vi "Configure Modulation(Phase).vi"(0 "VISA resource name":refnum<visa-resource-name>, 1 "Enable Phase Modulation (F: Disable)":bool, 2 "Phase Deviation (90 Degree)":dbl=90.0, 5 "Channel (1: Channel 1)":i32(ring)=1 items=["Channel 1"=1, "Channel 2"=2], 7 "PM Source (0: Internal)":i32(ring) items=["Internal", "External"], 9 "Modulation Waveform (0: Sinusoid)":i32(ring) items=["Sinusoid", "Square", "Triangle", "Ramp", "Nramp", "Noise", "User"], 11 "error in (no error)":errorcluster, 12 "Modulation Frequency (100 Hz)":dbl=100.0) -> (4 "VISA resource name out":refnum<visa-resource-name>, 15 "error out":errorcluster)   [LabVIEW 2012, in "RIGOL DG4000 Series.lvlib"]
doc: "Configures phase modulation."
uses:
  <instrlib>/RIGOL DG4000 Series/RIGOL DG4000 Series.lvlib
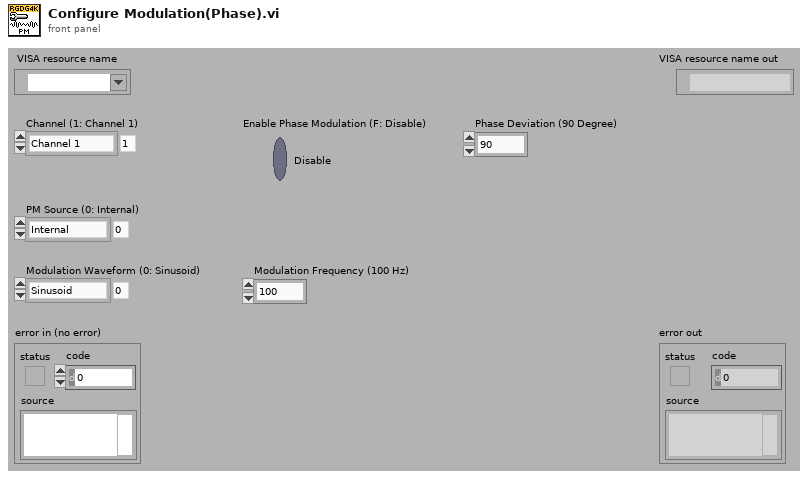
[diagram p1: front panel]
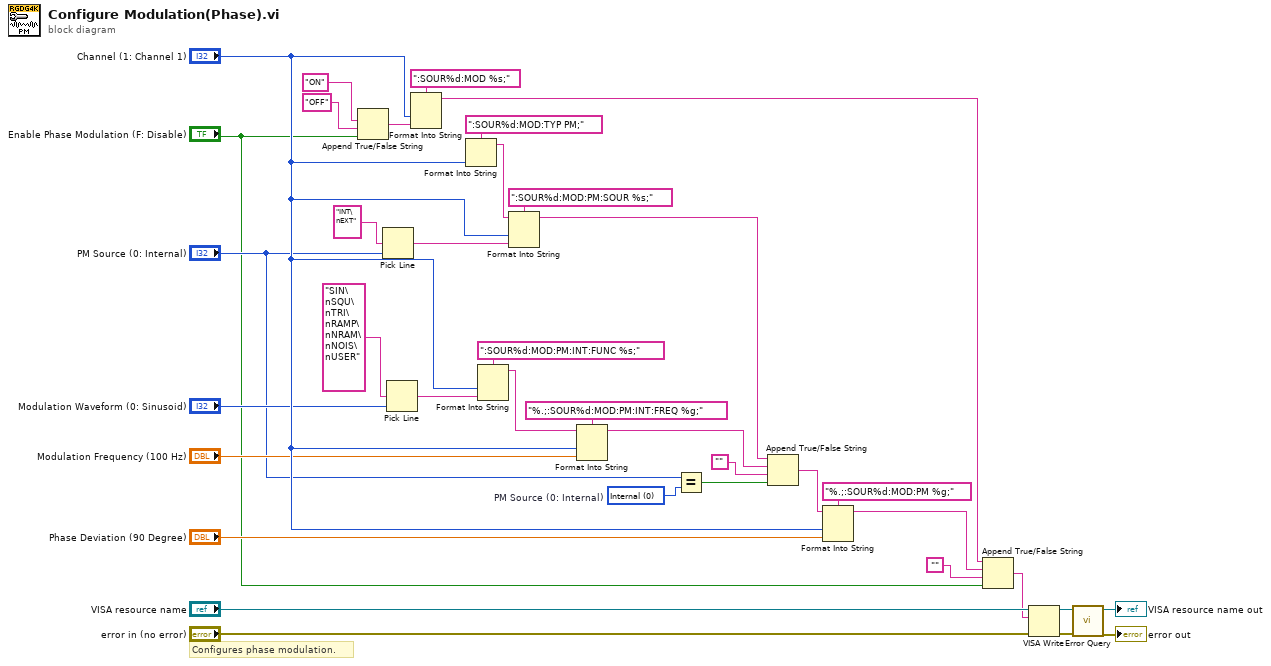
[diagram p0: block diagram]
diagram:
  w8 = 0 items=["Internal", "External"]  # PM Source (0: Internal)
  # "Configures phase modulation."
  n1 = Append True/False String(1:"Enable Phase Modulation (F: Disable)", 2:"OFF", 3:"ON") -> (0:w33:string)  [unwired: 1 out]
  n2 = Pick Line(multi-line string="INT\nEXT", line index="PM Source (0: Internal)") -> (output string=w28:string)  [unwired: 1 out]
  n3 = Pick Line(multi-line string="SIN\nSQU\nTRI\nRAMP\nNRAM\nNOIS\nUSER", line index="Modulation Waveform (0: Sinusoid)") -> (output string=w24:string)  [unwired: 1 out]
  n4 = Format Into String(format string=":SOUR%d:MOD %s;", "Channel (1: Channel 1)", w33) -> (resulting string=w2:string)  [unwired: 2 in, 1 out]
  n5 = Format Into String(format string=":SOUR%d:MOD:TYP PM;", "Channel (1: Channel 1)") -> (resulting string=w30:string)  [unwired: 2 in, 1 out]
  n6 = Format Into String(format string=":SOUR%d:MOD:PM:INT:FUNC %s;", "Channel (1: Channel 1)", w24) -> (resulting string=w23:string)  [unwired: 2 in, 1 out]
  n7 = Format Into String(format string=":SOUR%d:MOD:PM:SOUR %s;", initial string=w30, "Channel (1: Channel 1)", w28) -> (resulting string=w9:string)  [unwired: 1 in, 1 out]
  n8 = Format Into String(format string="%.;:SOUR%d:MOD:PM:INT:FREQ %g;", initial string=w23, "Channel (1: Channel 1)", "Modulation Frequency (100 Hz)") -> (resulting string=w10:string)  [unwired: 1 in, 1 out]
  n9 = Equal?(x="PM Source (0: Internal)", y=w8) -> (x = y?=w11:bool)
  n10 = Append True/False String(1:w11, 2:"", 3:w10, 4:w9) -> (0:w6:string)
  n11 = Format Into String(format string="%.;:SOUR%d:MOD:PM %g;", initial string=w6, "Channel (1: Channel 1)", "Phase Deviation (90 Degree)") -> (resulting string=w3:string)  [unwired: 1 in, 1 out]
  n12 = Append True/False String(1:"Enable Phase Modulation (F: Disable)", 2:"", 3:w3, 4:w2) -> (0:w4:string)
  n13 = VISA Write(VISA resource name="VISA resource name", write buffer=w4, error in (no error)="error in (no error)") -> (VISA resource name out=w16:refnum<visa-resource-name>, error out=w15:errorcluster)  [unwired: 1 out]
  n14 = call <instrlib>:"Error Query.vi"("error in (no error)"=w15, "VISA resource name"=w16) -> ("error out"=→"error out":errorcluster, "VISA resource name out"=→"VISA resource name out":refnum<visa-resource-name>)  [unwired: 8 out]
